vi "TestData_MySQL_Comm.vi"(8 "error in (no error)":errorcluster, 9 "Return Data (T)":bool=TRUE, 10 "Command Text":string="select column_name from information_schema.columns where table_schema='uel_te' and table_name='test_data'", 11 "ConnectionString":T1={"IP"="192.168.0.119", "Port"="3306", "DataBase"="uel_te", "User"="liguang", "Password"="123456"}) -> (0 "error out":errorcluster, 2 "Data":string[][](array[string])=[["ID"], ["name_pf"], ["name_ean13"], ["supplier_code"], ["date"], ["time"], ["operater_code"], ["sw_code"], ["sw_ver"], ["test_type"], ["item1_test"], ["item1_value"], ["item1_unit"], ["item1_limit_low"], ["item1_limit_high"], ["item2_test"], ["item2_value"], ["item2_unit"], ["item2_limit_low"], ["item2_limit_high"], ["item3_test"], ["item3_value"], ["item3_unit"], ["item3_limit_low"], ["item3_limit_high"], ["item4_test"], ["item4_value"], ["item4_unit"], ["item4_limit_low"], ["item4_limit_high"], ["item5_test"], ["item5_value"], ["item5_unit"], ["item5_limit_low"], ["item5_limit_high"], ["item6_test"], ["item6_value"], ["item6_unit"], ["item6_limit_low"], ["item6_limit_high"], ["item7_test"], ["item7_value"], ["item7_unit"], ["item7_limit_low"], ["item7_limit_high"], ["item8_test"], ["item8_value"], ["item8_unit"], ["item8_limit_low"], ["item8_limit_high"], ["item9_test"], ["item9_value"], ["item9_unit"], ["item9_limit_low"], ["item9_limit_high"], ["item10_test"], ["item10_value"], ["item10_unit"], ["item10_limit_low"], ["item10_limit_high"], ["item11_test"], ["item11_value"], ["item11_unit"], ["item11_limit_low"], ["item11_limit_high"], ["item12_test"], ["item12_value"], ["item12_unit"], ["item12_limit_low"], ["item12_limit_high"], ["item13_test"], ["item13_value"], ["item13_unit"], ["item13_limit_low"], ["item13_limit_high"], ["item14_test"], ["item14_value"], ["item14_unit"], ["item14_limit_low"], ["item14_limit_high"], ["item15_test"], ["item15_value"], ["item15_unit"], ["item15_limit_low"], ["item15_limit_high"], ["item16_test"], ["item16_value"], ["item16_unit"], ["item16_limit_low"], ["item16_limit_high"], ["item17_test"], ["item17_value"], ["item17_unit"], ["item17_limit_low"], ["item17_limit_high"], ["item18_test"], ["item18_value"], ["item18_unit"], ["item18_limit_low"], ["item18_limit_high"], ["item19_test"], ["item19_value"], ["item19_unit"], ["item19_limit_low"], ["item19_limit_high"], ["item20_test"], ["item20_value"], ["item20_unit"], ["item20_limit_low"], ["item20_limit_high"], ["item21_test"], ["item21_value"], ["item21_unit"], ["item21_limit_low"], ["item21_limit_high"], ["item22_test"], ["item22_value"], ["item22_unit"], ["item22_limit_low"], ["item22_limit_high"], ["item23_test"], ["item23_value"], ["item23_unit"], ["item23_limit_low"], ["item23_limit_high"], ["item24_test"], ["item24_value"], ["item24_unit"], ["item24_limit_low"], ["item24_limit_high"], ["item25_test"], ["item25_value"], ["item25_unit"], ["item25_limit_low"], ["item25_limit_high"], ["item26_test"], ["item26_value"], ["item26_unit"], ["item26_limit_low"], ["item26_limit_high"], ["item27_test"], ["item27_value"], ["item27_unit"], ["item27_limit_low"], ["item27_limit_high"], ["item28_test"], ["item28_value"], ["item28_unit"], ["item28_limit_low"], ["item28_limit_high"], ["item29_test"], ["item29_value"], ["item29_unit"], ["item29_limit_low"], ["item29_limit_high"], ["item30_test"], ["item30_value"], ["item30_unit"], ["item30_limit_low"], ["item30_limit_high"], ["item31_test"], ["item31_value"], ["item31_unit"], ["item31_limit_low"], ["item31_limit_high"], ["item32_test"], ["item32_value"], ["item32_unit"], ["item32_limit_low"], ["item32_limit_high"], ["item33_test"], ["item33_value"], ["item33_unit"], ["item33_limit_low"], ["item33_limit_high"], ["item34_test"], ["item34_value"], ["item34_unit"], ["item34_limit_low"], ["item34_limit_high"], ["item35_test"], ["item35_value"], ["item35_unit"], ["item35_limit_low"], ["item35_limit_high"], ["item36_test"], ["item36_value"], ["item36_unit"], ["item36_limit_low"], ["item36_limit_high"], ["item37_test"], ["item37_value"], ["item37_unit"], ["item37_limit_low"], ["item37_limit_high"], ["item38_test"], ["item38_value"], ["item38_unit"], ["item38_limit_low"], ["item38_limit_high"], ["item39_test"], ["item39_value"], ["item39_unit"], ["item39_limit_low"], ["item39_limit_high"], ["item40_test"], ["item40_value"], ["item40_unit"], ["item40_limit_low"], ["item40_limit_high"], ["item41_test"], ["item41_value"], ["item41_unit"], ["item41_limit_low"], ["item41_limit_high"], ["item42_test"], ["item42_value"], ["item42_unit"], ["item42_limit_low"], ["item42_limit_high"], ["item43_test"], ["item43_value"], ["item43_unit"], ["item43_limit_low"], ["item43_limit_high"], ["item44_test"], ["item44_value"], ["item44_unit"], ["item44_limit_low"], ["item44_limit_high"], ["item45_test"], ["item45_value"], ["item45_unit"], ["item45_limit_low"], ["item45_limit_high"], ["item46_test"], ["item46_value"], ["item46_unit"], ["item46_limit_low"], ["item46_limit_high"], ["item47_test"], ["item47_value"], ["item47_unit"], ["item47_limit_low"], ["item47_limit_high"], ["spare1"], ["spare2"], ["spare3"], ["spare4"], ["jig_code"], ["total_qty"], ["field_code"], ["spare5"], ["test_time"], ["test_result"], ["serial_number"]])   [LabVIEW 2012, in "Lib_UEL.ATE.lvlib" / "Lib_TestData.lvlib"]
uses:
  Lib_TestData.lvlib
panel:
  out "MaxRecords":i32
  out "RecordSet":refnum<k7>
  out "Rows Affected":i32
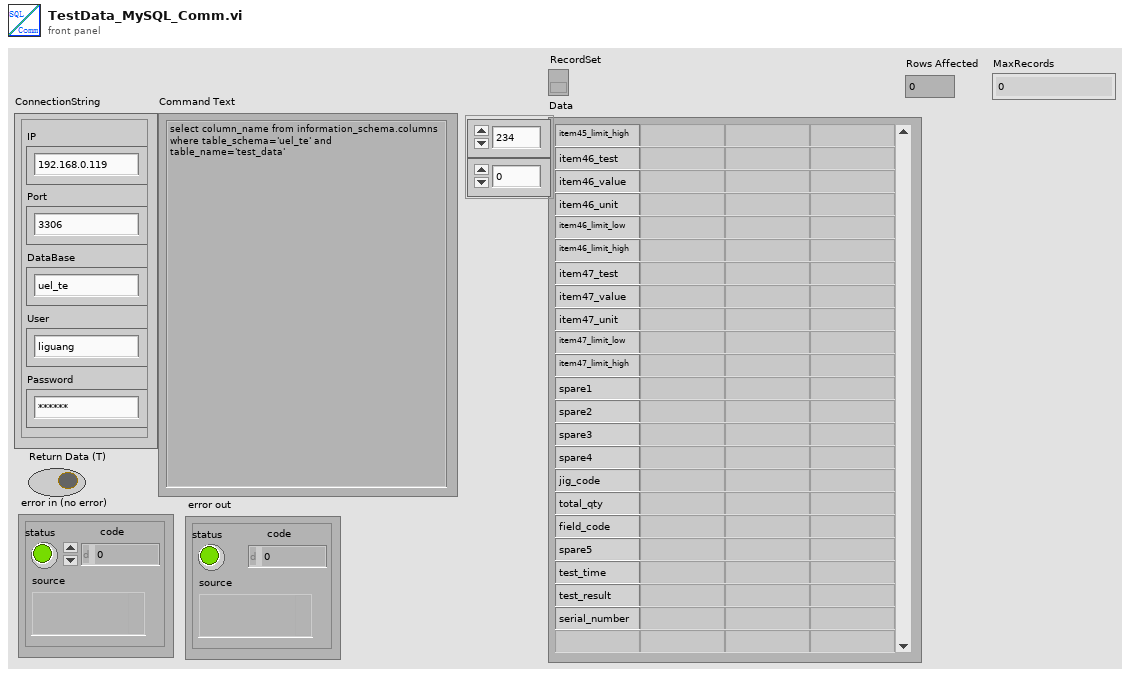
[diagram p1: front panel]
types:
  T1 = cluster{"IP":string, "Port":string, "DataBase":string, "User":string, "Password":string}
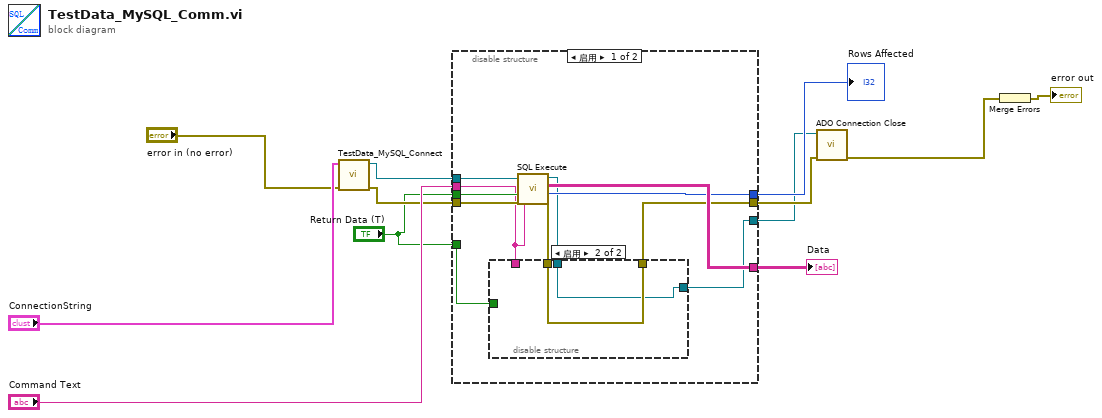
[diagram p0: block diagram]
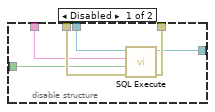
[diagram p2: hidden frame]
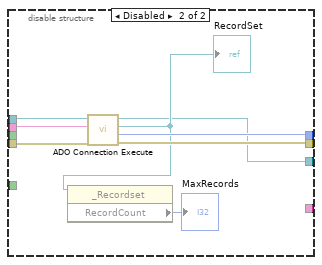
[diagram p3: hidden frame]
diagram:
  n1 = call "TestData_MySQL_Connect.vi"("error in (no error)"="error in (no error)", "ConnectionString"="ConnectionString") -> ("Error Out"=w9:errorcluster, "Connection Out"=w8:refnum<k7>)  [unwired: 8 in]
  n2 = disable-structure shown="启用" {
    disable-tunnel: [w16 w36] -> w3
    disable-tunnel: "Command Text" -> [w14 w37]
    disable-tunnel: "Return Data (T)" -> [w23 _]
    disable-tunnel: w9 -> [w22 w38]
    disable-tunnel: w8 -> [w21 w39]
    disable-tunnel: [w20 _] -> w7
    disable-tunnel: [w19 w35] -> w6
    disable-tunnel: [w15 w32] -> w1
    disable-tunnel: "Return Data (T)" -> [w13 _]
    frame Enabled {
      n3 = call <userlib>:"SQL Execute.vi"("error in (no error)"=w22, "Return Data (T)"=w23, "Command Text"=w14, "ADODB._Connection In"=w21) -> ("error out"=w17:errorcluster, "Rows Affected"=w19:i32, "Data"=w20:string[][], "ADODB._Connection Out"=w18:refnum<k7>)  [unwired: 4 in]
      n4 = disable-structure shown="启用" {
        disable-tunnel: w18 -> [w29 w30]
        disable-tunnel: w17 -> [w28 w31]
        disable-tunnel: [w27 w31] -> w16
        disable-tunnel: [w26 w30] -> w15
        disable-tunnel: w14 -> [w25 _]
        disable-tunnel: w13 -> [w24 _]
        frame Disabled {
          n5 = call <userlib>:"SQL Execute.vi"("error in (no error)"=w28, "Return Data (T)"=w24, "Command Text"=w25, "ADODB._Connection In"=w29) -> ("error out"=w27:errorcluster, "ADODB._Connection Out"=w26:refnum<k7>)  [unwired: 4 in, 2 out]
        }
        frame Enabled {
        }
      }
    }
    frame Disabled {
      n6 = call <userlib>:"ADO Connection Execute.vi"("error in (no error)"=w38, "CommandText"=w37, "ADODB._Connection In"=w39) -> ("error out"=w36:errorcluster, "RecordsAffected"=w35:i32, "RecordSet"=w33:refnum<k7>, "ADODB._Connection Out"=w32:refnum<k7>)  [unwired: 5 in]
      "RecordSet" <- w33
      n7 = property class="_Recordset"(reference=w33) -> ("RecordCount"=→"MaxRecords":i32)  [unwired: 1 in, 2 out]
    }
  }
  "Data" <- w7
  "Rows Affected" <- w6
  n8 = call <userlib>:"ADO Connection Close.vi"("error in (no error)"=w3, "ADODB._Connection In"=w1) -> ("error out"=w5:errorcluster)  [unwired: 8 in, 1 out]
  n9 = Merge Errors(w5) -> (→"error out":errorcluster)
